vi "Determine Warnings Error (4-1).vi"(8 "error in (no error)":errorcluster, 9 "Min Temp":dbl, 10 "Max Temp":dbl, 11 "Current Temp":dbl) -> (0 "error out":errorcluster, 1 "Warning?":bool, 2 "Warning Text":string)   [LabVIEW 2014]
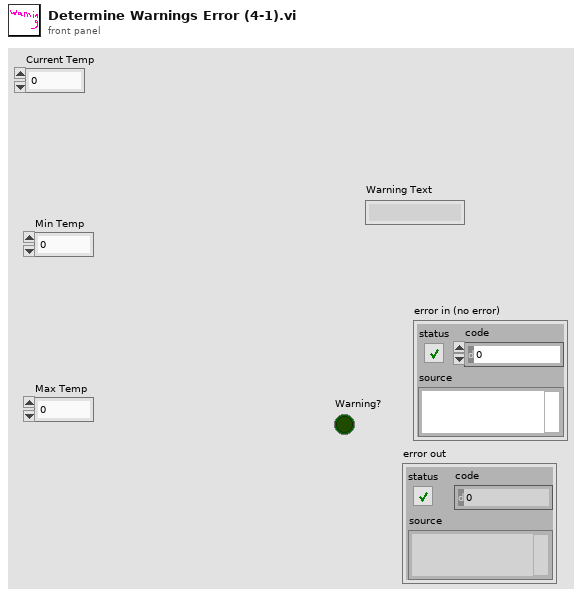
[diagram p1: front panel]
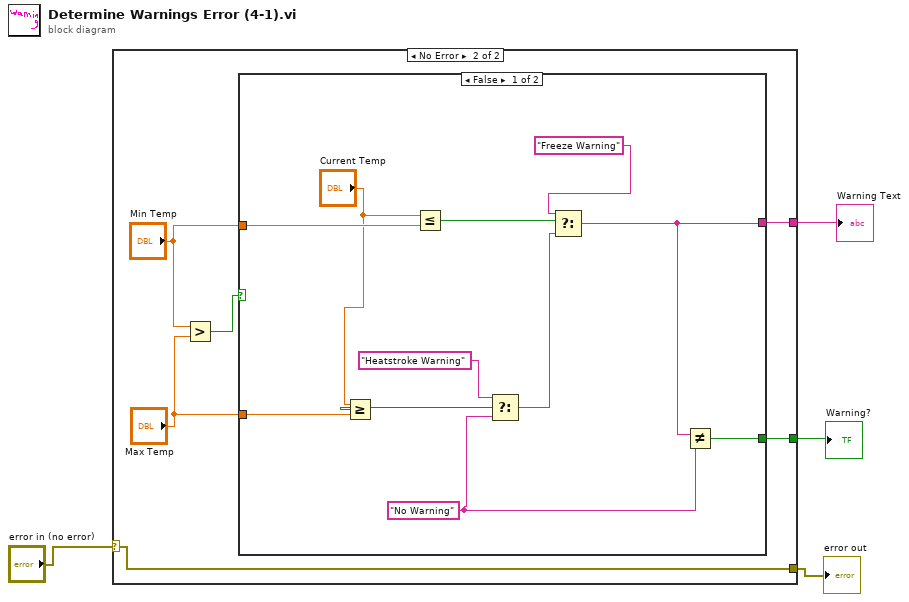
[diagram p0: block diagram]
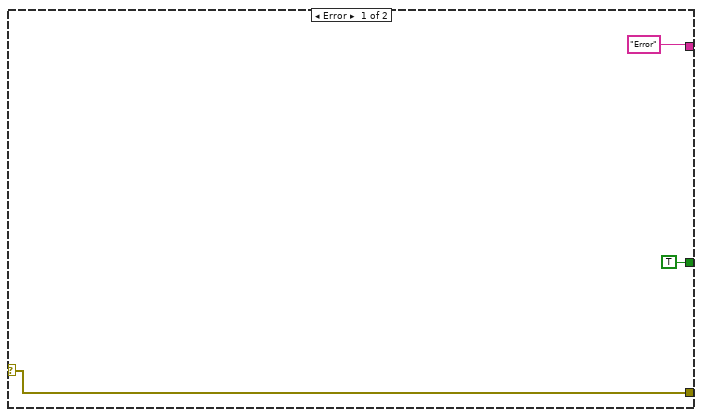
[diagram p2: hidden frame]
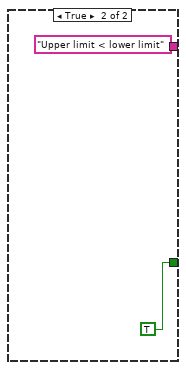
[diagram p3: hidden frame]
diagram:
  n1 = case shown="No Error" "error in (no error)" {
    selector: "error in (no error)" -> [w5 w8]
    tunnel: ["Error" w13] -> w4
    tunnel: [TRUE ("Warning?") w9] -> w3
    tunnel: [w5 w8] -> w2
    frame Error {
    }
    frame No Error {
      n2 = Greater?(x="Min Temp", y="Max Temp") -> (0:w10:bool)
      n3 = case shown="False" w10 {
        tunnel: "Min Temp" -> [w24 _]
        tunnel: "Max Temp" -> [w23 _]
        tunnel: [w15 "Upper limit < lower limit"] -> w13
        tunnel: [w14 TRUE ("Warning?")] -> w9
        frame False {
          w16 = "No Warning"
          n4 = Greater Or Equal?(x="Current Temp", y=w23) -> (x >= y?=w21:bool)
          n5 = Less Or Equal?(x="Current Temp", y=w24) -> (x <= y?=w19:bool)
          n6 = Select(t="Heatstroke Warning", s=w21, f=w16) -> (s? t:f=w17:string)
          n7 = Select(t="Freeze Warning", s=w19, f=w17) -> (s? t:f=w15:string)
          n8 = Not Equal?(x=w15, y=w16) -> (x != y?=w14:bool)
        }
        frame True {
        }
      }
    }
  }
  "Warning Text" <- w4
  "Warning?" <- w3
  "error out" <- w2
